vi "PCO_Create_Metadata_File.vi"(8 "entrée d'erreur":errorcluster, 11 "PCO_Config":T1={"Exposure time (s)"=0.01, "TriggerMode"=0, "ROI X0"=1, "ROI Y0"=1, "ROI X1"=2048, "ROI Y1"=2048, "Binning"=1} {"TriggerMode" items=["auto sequence", "software trigger", "external exposure start", "external exposure control"]}) -> (0 "sortie d'erreur":errorcluster)   [LabVIEW 2026]
uses:
  Controls/PCO_Config.ctl
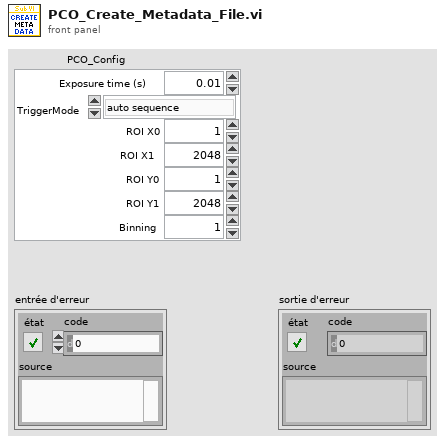
[diagram p1: front panel]
types:
  T1 = typedef "PCO_Config.ctl" = cluster{"Exposure time (s)":dbl, "TriggerMode":u16, "ROI X0":u16, "ROI Y0":u16, "ROI X1":u16, "ROI Y1":u16, "Binning":u8}
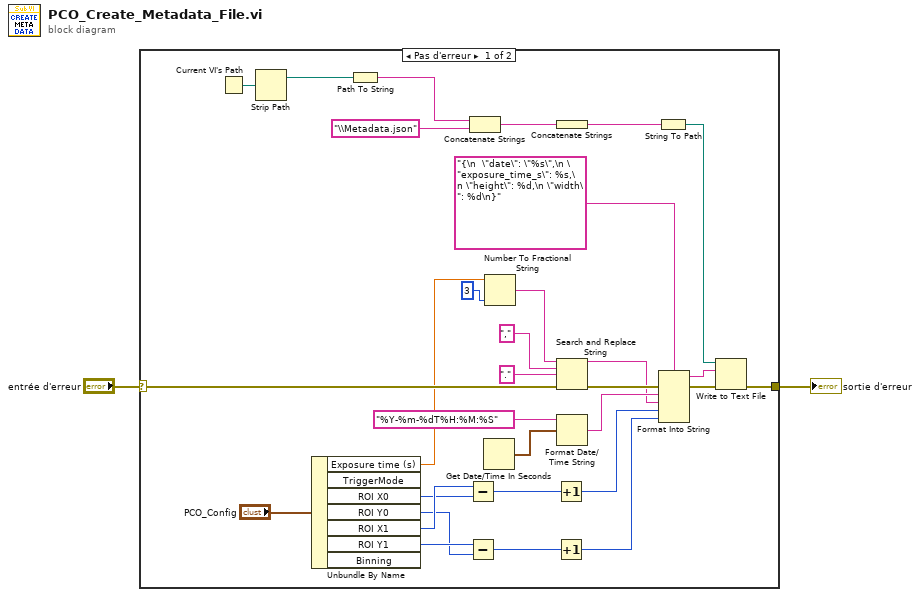
[diagram p0: block diagram]
diagram:
  n1 = case shown="Pas d'erreur" "entrée d'erreur" {
    selector: "entrée d'erreur" -> [w22 w34]
    tunnel: [w24 w34] -> w2
    frame No Error {
      n2 = Current VI's Path() -> (path=w30:path)
      n3 = Strip Path(path=w30) -> (stripped path=w29:path)  [unwired: 1 out]
      n4 = Unbundle By Name("PCO_Config") -> ("Exposure time (s)"=w12:dbl, "ROI X0"=w9:u16, "ROI Y0"=w4:u16, "ROI X1"=w10:u16, "ROI Y1"=w5:u16)  [unwired: 2 out]
      n5 = Path To String(path=w29) -> (string=w32:string)
      n6 = Subtract(x=w10, y=w9) -> (x-y=w8:u16)
      n7 = Subtract(x=w5, y=w4) -> (x-y=w6:u16)
      n8 = Concatenate Strings(w32, "\\Metadata.json" ("chaîne")) -> (w31:string)
      n9 = Get Date/Time In Seconds() -> (seconds since 1Jan1904=w16:timestamp)
      n10 = Number To Fractional String(number=w12, precision (6)=i16 3 ("précision (6)")) -> (F-format string=w20:string)  [unwired: 2 in]
      n11 = Increment(x=w8) -> (x+1=w7:u16)
      n12 = Increment(x=w6) -> (x+1=w3:u16)
      n13 = Concatenate Strings(w31) -> (w26:string)
      n14 = Search and Replace String(input string=w20, search string="," ("chaîne recherchée"), replace string="." ("chaîne de remplacement (\"\")"), error in=w22) -> (result string=w11:string, error out=w21:errorcluster)  [unwired: 4 in, 2 out]
      n15 = Format Date/Time String(time format string (%c)="%Y-%m-%dT%H:%M:%S" ("chaîne de format de l'heure (%c)"), seconds (now)=w16) -> (date/time string=w14:string)  [unwired: 1 in]
      n16 = String To Path(string=w26) -> (path=w25:path)
      n17 = Format Into String(format string="{\n  \"date\": \"%s\",\n \"exposure_time_s\": %s,\n \"height\": %d,\n \"width\": %d\n}" ("chaîne de format"), error in=w21, w14, w11, w7, w3) -> (resulting string=w27:string, error out=w23:errorcluster)  [unwired: 1 in]
      n18 = Write to Text File(file (use dialog)=w25, text=w27, error in=w23) -> (error out=w24:errorcluster)  [unwired: 1 in, 2 out]
    }
    frame Error {
    }
  }
  "sortie d'erreur" <- w2
